vi "ToolBarButtonDraw_ZoomWindow.vi"(6 "Color":u32(colorbox), 10 "rect":T1, 11 "Pict IN":picture) -> (3 "Pict OUT":picture)   [LabVIEW 2020, in "Sgraph_lib_V1.lvlib" / "Gviewer.lvclass"]
doc: "Draw Focus icon in button bar"
uses:
  Gviewer.lvclass
  <vilib>/picture/picture.llb/imagedata.ctl
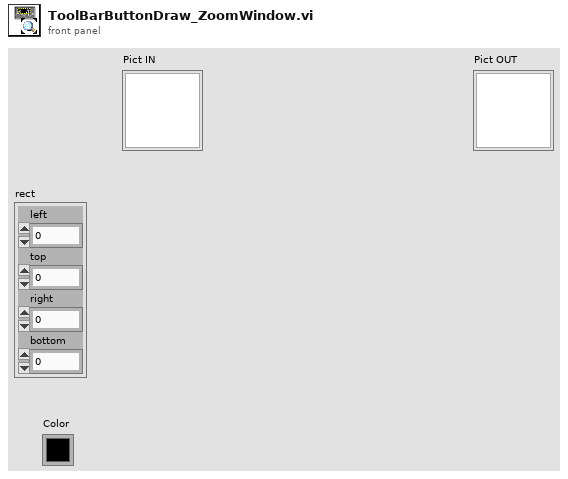
[diagram p1: front panel]
types:
  T1 = cluster{"left":i16, "top":i16, "right":i16, "bottom":i16}
  T2 = typedef "imagedata.ctl" = cluster{"image type":i32, "image depth":i32, "image":u8[], "mask":u8[], "colors":u32[], "Rectangle":cluster{"left":i16, "top":i16, "right":i16, "bottom":i16}}
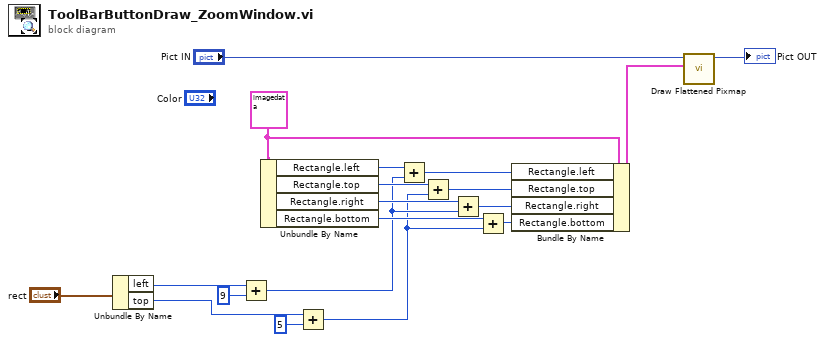
[diagram p0: block diagram]
diagram:
  w8 = T2 {"image type"=0, "image depth"=24, "image"=array[1170 elements], "mask"=[], "colors"=[], "Rectangle"={"left"=0, "top"=0, "right"=26, "bottom"=15}} ("image data")
  n1 = Unbundle By Name("rect") -> ("left"=w12:i16, "top"=w10:i16)
  n2 = Add(x=w12, y=i16 9) -> (x+y=w11:i16)
  n3 = Unbundle By Name(w8) -> ("Rectangle.left"=w16:i16, "Rectangle.top"=w15:i16, "Rectangle.right"=w14:i16, "Rectangle.bottom"=w13:i16)
  n4 = Add(x=w10, y=i16 5) -> (x+y=w9:i16)
  n5 = Add(x=w16, y=w11) -> (x+y=w4:i16)
  n6 = Add(x=w15, y=w9) -> (x+y=w5:i16)
  n7 = Add(x=w14, y=w11) -> (x+y=w6:i16)
  n8 = Add(x=w13, y=w9) -> (x+y=w7:i16)
  n9 = Bundle By Name(cluster=w8, "Rectangle.left"=w4, "Rectangle.top"=w5, "Rectangle.right"=w6, "Rectangle.bottom"=w7) -> (w3:T2)
  n10 = call <vilib>:"Draw Flattened Pixmap.vi"("image data"=w3, "picture"="Pict IN") -> ("new picture"=→"Pict OUT":picture)  [unwired: 7 in]
